vi "未命名 1.vi"(9 "Reference data in":cluster{"参考值":dbl, "参考值时间":timestamp}[](array[cluster]), 10 "Para":T2, 11 "data in":cluster{"数值":dbl, "时间标识":timestamp}) -> (1 "Reference data out":cluster{"参考值":dbl, "参考值时间":timestamp}[](array[cluster]), 3 "data out":T1)   [LabVIEW 2016]
uses:
  <vilib>/Analysis/NI_AALBase.lvlib
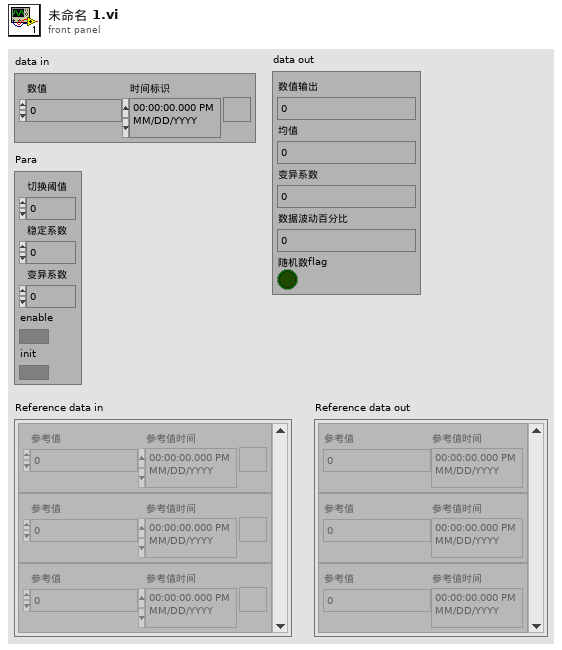
[diagram p1: front panel]
types:
  T1 = cluster{"数值输出":dbl, "均值":dbl, "变异系数":dbl, "数据波动百分比":dbl, "随机数flag":bool}
  T2 = cluster{"切换阈值":dbl, "稳定系数":dbl, "变异系数":dbl, "enable":bool, "init":bool}
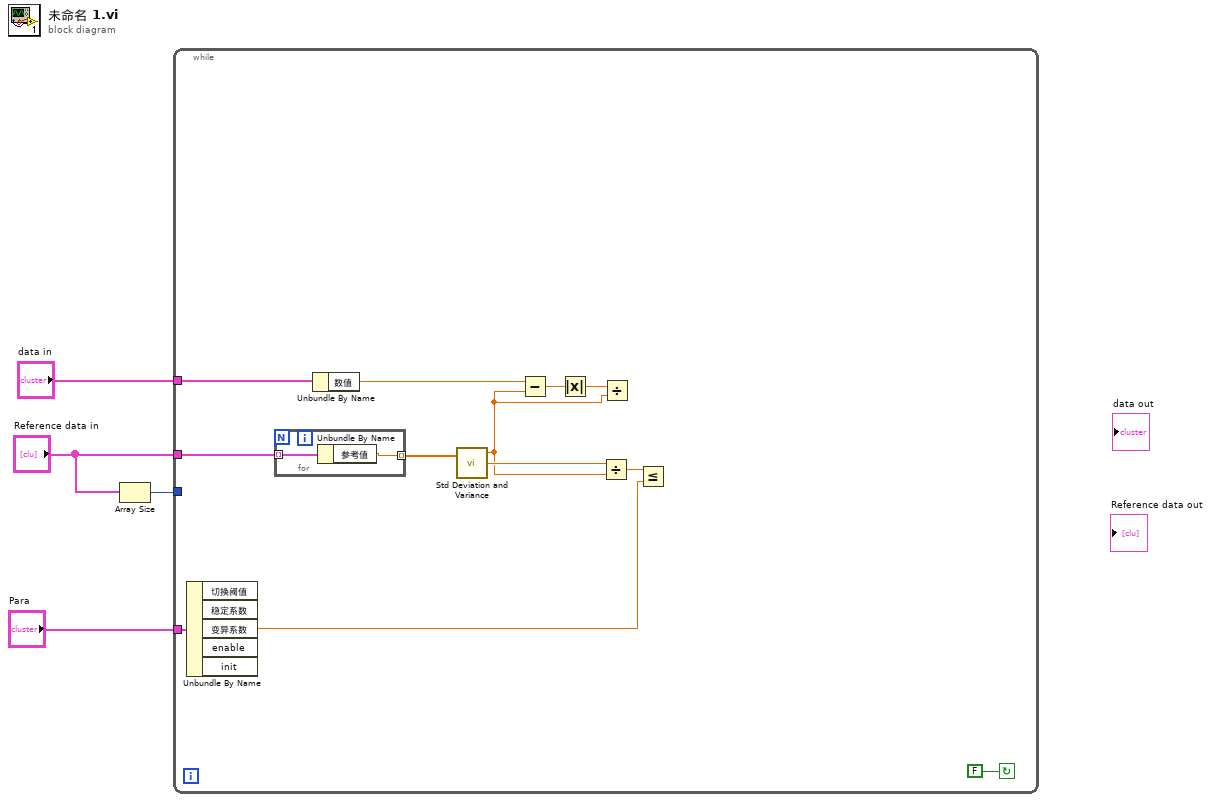
[diagram p0: block diagram]
diagram:
  n1 = Array Size(array="Reference data in") -> (size(s)=w1:i32)
  n2 = while {
    tunnel: "data in" -> [w11]
    tunnel: "Reference data in" -> [w14]
    tunnel: "Para" -> [w15]
    tunnel: w1 -> [_]
    stop <- FALSE continue-if-true
    n3 = Unbundle By Name(w15) -> ("变异系数"=w5:dbl)  [unwired: 4 out]
    n4 = for {
      tunnel: w14 -> [w18] mode=indexing
      tunnel: [w17] -> w13 mode=indexing
      n5 = Unbundle By Name(w18) -> ("参考值"=w17:dbl)
    }
    n6 = Unbundle By Name(w11) -> ("数值"=w10:dbl)
    n7 = call <vilib>:"Std Deviation and Variance.vi"("X"=w13) -> ("mean"=w7:dbl, "standard deviation"=w12:dbl)  [unwired: 1 in, 1 out]
    n8 = Subtract(x=w10, y=w7) -> (x-y=w9:dbl)
    n9 = Absolute Value(x=w9) -> (abs(x)=w8:dbl)
    n10 = Divide(x=w12, y=w7) -> (x/y=w6:dbl)
    n11 = Divide(x=w8, y=w7) -> ()  [unwired: 1 out]
    n12 = Less Or Equal?(x=w6, y=w5) -> ()  [unwired: 1 out]
  }
